vi "TestDAQOrcaFlash.vi"   [LabVIEW 2012]
uses:
  DAQOrcaFlash/DAQOrcaFlash.lvclass
  Murmex/LabVIEW/Murmex/Murmex/Murmex.lvclass
panel:
  # "Test DAQ"
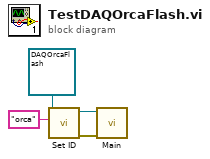
[diagram p0: block diagram]
diagram:
  n1 = call "Set ID.vi"("id"="orca", "Murmex in"=refnum<class "DAQOrcaFlash.lvclass"> refnum ("DAQOrcaFlash.lvclass")) -> ("error out"=w4:errorcluster, "Murmex out"=w1:refnum<class "DAQOrcaFlash.lvclass">)  [unwired: 8 in]
  n2 = call-dynamic "Main.vi"("error in (no error)"=w4, "DAQMH121119OrcaFlashBase in"=w1) -> ()  [unwired: 8 in, 2 out]
